vi "zmq_recv.vi"(5 "no block? (F)":bool, 6 "error in":errorcluster, 9 "socket in":refnum<class "zmq_socket.lvclass">) -> (0 "error out":errorcluster, 1 "more?":bool, 2 "data":string, 3 "socket out":refnum<class "zmq_socket.lvclass">, 4 "timeout?":bool)   [LabVIEW 2019, in "zeromq.lvlib" / "zmq_socket.lvclass"]
doc: "Receive a message from the socket and returns the received data as a LabVIEW string (which may contain NULL). If receiving a multi-part message, this VI must be called for each part of the message, and it is the user's obligation to check if this is required. Alternatively, use the zmq_recv_multi VI, which handles this automatically.\n\nIf <b>no block?</b> is True, the function call will return immediately. Use zmq_check_timeout to see if it was simply a timeout or an error occurred.\n\nOtherwise this call will block until a message is received, an error is raised, or the socket is closed.\n\nDetailed API documentation: http://api.zeromq.org/3-2:zmq-recv"
uses:
  zmq_socket.lvclass
  zmq_socket.lvclass/zmq_socket.ctl
  <vilib>/Utility/error.llb/Error Cluster From Error Code.vi
  zeromq.lvlib
panel:
  # "ØMQ"
  # "labview"
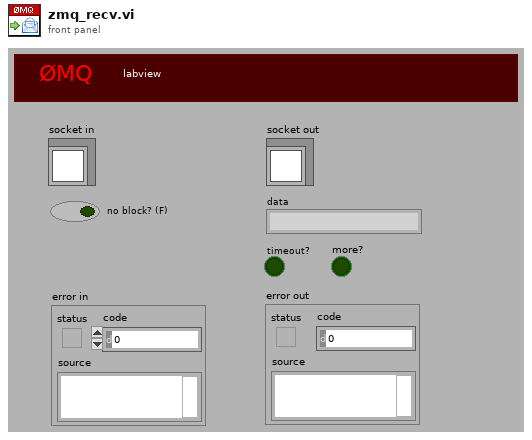
[diagram p1: front panel]
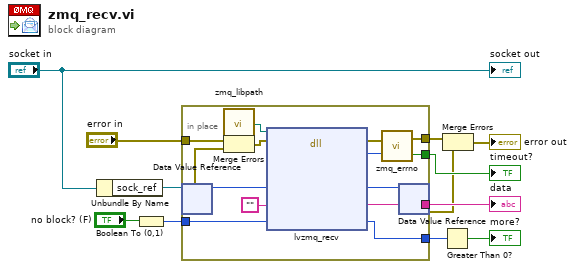
[diagram p0: block diagram]
diagram:
  n1 = Unbundle By Name("socket in") -> ("sock_ref"=w4:refnum<data-value>)
  n2 = Boolean To (0,1)(Boolean="no block? (F)") -> (0, 1=w11:i16)
  n3 = in-place {
    in-place-border: [w24] -> w12
    in-place-border: w11 -> [w23]
    in-place-border: [w22] -> w3
    in-place-border: "error in" -> [w21]
    in-place-border: [w20] -> w8
    in-place-border: [w19] -> w7
    n4 = in-place-dvr #1(w4) -> (w18:u64, w13:errorcluster)
    n5 = call "zmq_libpath.vi"() -> ("path"=w15:path)
    n6 = Merge Errors(w21, w13) -> (w14:errorcluster)
    n7 = dll-call lib="?" fn="lvzmq_recv" ("zmq_labview.dll:lvzmq_socket")(path in=w15, error in=w14, "sock_obj"=w18, "data"="", "flags"=w23) -> (error out=w26:errorcluster, "return type"=w25:i32, "sock_obj"=w17:u64, "data"=w22:string, "flags"=w19:i32)  [unwired: 3 in, 1 out]
    n8 = call "zmq_errno.vi"("retval"=w25, "error in"=w26) -> ("again?"=w24:bool, "error out"=w20:errorcluster)
    n9 = in-place-dvr #1(w17) -> (w1:errorcluster)  [unwired: 1 out]
  }
  "data" <- w3
  "timeout?" <- w12
  n10 = Greater Than 0?(x=w7) -> (x > 0?=→"more?":bool)
  n11 = Merge Errors(w8, w1) -> (→"error out":errorcluster)
  "socket out" <- "socket in"
